vi "read_sub_pend.vi"(10 "instance":i32) -> (0 "Txlat_ms":dbl, 1 "Pendulum ENC 2":i32, 2 "ENC VEL 1":dbl, 3 "ENC POS 1":i32)   [LabVIEW 2024]
uses:
  SADI_Pendulum_lib/pendulumApp.lvlib
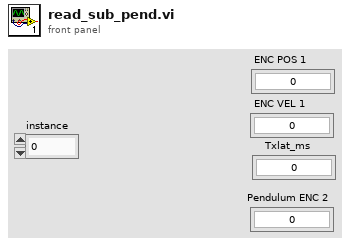
[diagram p1: front panel]
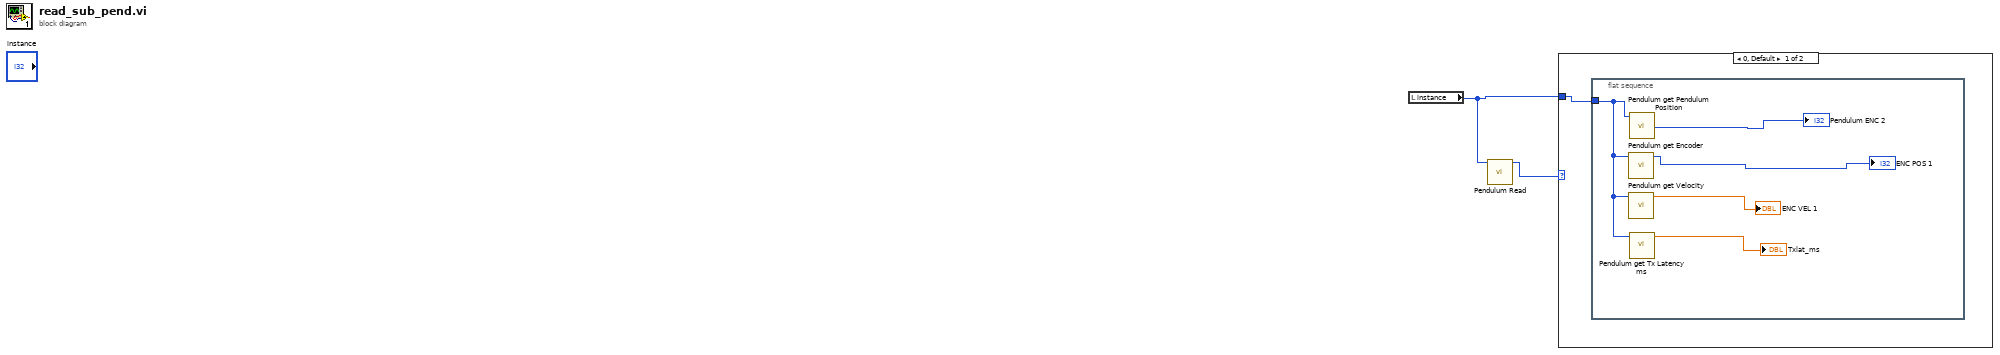
[diagram p0: block diagram]
diagram:
  n1 = local read "instance"() -> (w2:i32)
  n2 = call "Pendulum Read.vi"("instance"=w2) -> ("function return"=w1:i32)  [unwired: 10 in]
  n3 = case shown="0, Default" w1 {
    tunnel: w2 -> [w3 _]
    frame 0, Default {
      n4 = flat-sequence {
        tunnel: w3 -> [w6]
        frame #0 {
          n5 = call "Pendulum get Encoder.vi"("instance"=w6) -> ("function return"=→"ENC POS 1":i32)  [unwired: 10 in]
          n6 = call "Pendulum get Velocity.vi"("instance"=w6) -> ("function return"=→"ENC VEL 1":dbl)  [unwired: 10 in]
          n7 = call "Pendulum get Pendulum Position.vi"("instance"=w6) -> ("function return"=→"Pendulum ENC 2":i32)  [unwired: 10 in]
          n8 = call "Pendulum get Tx Latency ms.vi"("instance"=w6) -> ("function return"=→"Txlat_ms":dbl)  [unwired: 10 in]
        }
      }
    }
    frame 1 {
    }
  }
